vi "aal_moving average with decimation by order.vi"   [LabVIEW 2010, in "NI_AALPro.lvlib"]
uses:
  NI_AALPro.lvlib
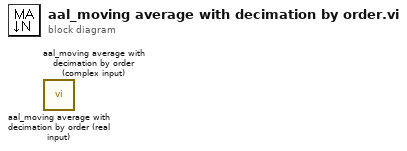
[diagram p0: block diagram]
diagram:
  n1 = call "aal_moving average with decimation by order (real input).vi"() -> ()  [unwired: 3 in, 1 out]
  n2 = call "aal_moving average with decimation by order (complex input).vi"() -> ()  [unwired: 3 in, 1 out]
